vi "PV ActiveLine - SetPoint.vi"(0 "Referenz in":refnum<visa-resource-name>, 1 "Setpoint":i32(ring) items=["SP 1", "SP 2", "SP 3", "SP 4"], 2 "W/R":bool, 5 "Channel Nr.":i32(ring) items=["Turned off", "Turned on", "Measurement channel 1", "Measurement channel 2"], 7 "Setpoint low":dbl=1000.0 min=0.0 max=41000.0 format="%.2e", 9 "Setpoint high":dbl=1100.0 min=0.0 max=41000.0 format="%.2e", 11 "Fehler (Eingang)":errorcluster) -> (4 "Referenz out":refnum<visa-resource-name>, 6 "Get Channel Nr":i32(ring) items=["Turned off", "Turned on", "Measurement channel 1", "Measurement channel 2"], 8 "Get Setpoint low":dbl min=0.0 max=41000.0 format="%.2e", 10 "Get Setpoint high":dbl min=0.0 max=41000.0 format="%.2e", 15 "Cluster (Ausgang)":errorcluster)   [LabVIEW 2013, in "PV ActiveLine.lvlib"]
doc: "SPx - Threshold Value Setting, Allocation\n\nTransmit: SPx [,a,x.xxxxEsxx,y.yyyyEsyy]\nReceive: a,x.xxxxEsxx,y.yyyyEsyy\n\nSwitching function, x =\n1 –> Switching function 1\n2 –> Switching function 2\n3 –> Switching function 3\n4 –> Switching function 4\na Switching function assignment, a =\n0 –> Turned off\n1 –> Turned on\n2 –> Measurement channel 1\n3 –> Measurement channel 2\nx.xxxxEsxx Lower threshold 1) [in current pressure unit]\n(default = depending on gauge)\ny.yyyyEsyy Upper threshold 1) [in current pressure unit]\n(default = depending on gauge)"
uses:
  <instrlib>/PV ActiveLine/PV ActiveLine.lvlib
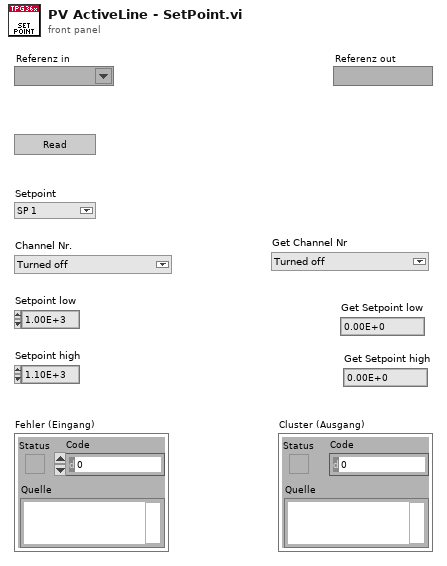
[diagram p1: front panel]
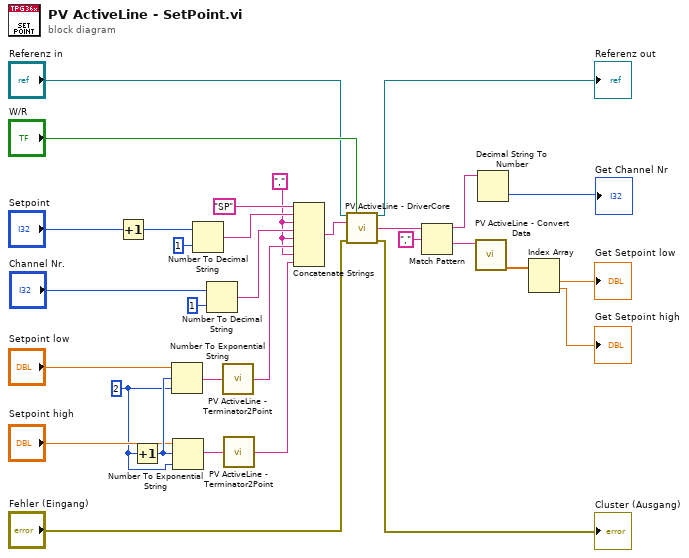
[diagram p0: block diagram]
diagram:
  w1 = u8 2 ("Kommastellen")
  w5 = "," ("Command")
  n1 = Increment(x="Setpoint") -> (x+1=w30:i32)
  n2 = Increment(x=w1) -> (x+1=w7:u8)
  n3 = Number To Exponential String(number="Setpoint low", precision (6)=w1, 3:w7) -> (E-format string=w9:string)  [unwired: 1 in]
  n4 = Number To Exponential String(number="Setpoint high", precision (6)=w1, 3:w7) -> (E-format string=w8:string)  [unwired: 1 in]
  n5 = Number To Decimal String(number=w30, width (-)=i16 1) -> (decimal integer string=w24:string)
  n6 = Number To Decimal String(number="Channel Nr.", width (-)=i16 1) -> (decimal integer string=w25:string)
  n7 = call <instrlib>:"PV ActiveLine - Terminator2Point.vi"("Eingangstring"=w9) -> ("Ausgangstring"=w6:string)
  n8 = call <instrlib>:"PV ActiveLine - Terminator2Point.vi"("Eingangstring"=w8) -> ("Ausgangstring"=w4:string)
  n9 = Concatenate Strings("SP" ("Command"), w24, w5, w25, w5, w6, w5, w4) -> (w21:string)
  n10 = call <instrlib>:"PV ActiveLine - DriverCore.vi"("Referenz in"="Referenz in", "Write/Read"="W/R", "Command"=w21, "Fehler (Eingang)"="Fehler (Eingang)") -> ("Referenz out"=→"Referenz out":refnum<visa-resource-name>, "String Out"=w16:string, "Cluster (Ausgang)"=→"Cluster (Ausgang)":errorcluster)  [unwired: 9 in]
  n11 = Match Pattern(string=w16, regular expression=",") -> (before substring=w22:string, after substring=w13:string)  [unwired: 1 in, 2 out]
  n12 = call <instrlib>:"PV ActiveLine - Convert Data.vi"("String in"=w13) -> ("DBL out"=w12:dbl[])  [unwired: 7 in, 3 out]
  n13 = Decimal String To Number(string=w22) -> (number=→"Get Channel Nr":i32)  [unwired: 2 in, 1 out]
  n14 = Index Array(array=w12) -> (element #1=→"Get Setpoint low":dbl, element #2=→"Get Setpoint high":dbl)  [unwired: 2 in]
